vi "Set Inertia Matrix as 1D Array.vi"(8 "error in (no error)":errorcluster, 10 "Inertia":dbl[](array[numeric]), 11 "Link in":refnum<class "Link.lvclass">) -> (0 "error out":errorcluster, 3 "Link out":refnum<class "Link.lvclass">)   [LabVIEW 2013, in "Link.lvclass"]
uses:
  Link.lvclass
  Link.lvclass/Link.ctl
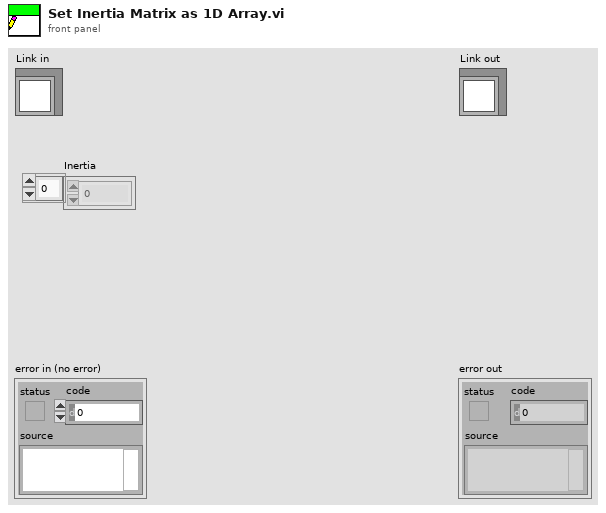
[diagram p1: front panel]
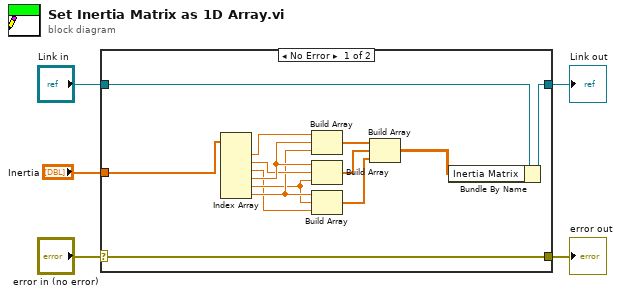
[diagram p0: block diagram]
diagram:
  n1 = case shown="No Error" "error in (no error)" {
    selector: "error in (no error)" -> [w19 w20]
    tunnel: [w19 w20] -> w4
    tunnel: [w17 w21] -> w2
    tunnel: "Link in" -> [w18 w21]
    tunnel: "Inertia" -> [w7 _]
    frame No Error {
      n2 = Index Array(array=w7) -> (element #1=w16:dbl, element #2=w14:dbl, element #3=w11:dbl, element #4=w15:dbl, element #5=w12:dbl, element #6=w13:dbl)  [unwired: 6 in]
      n3 = Build Array(w16, w15, w13) -> (w10:dbl[])
      n4 = Build Array(w15, w14, w12) -> (w9:dbl[])
      n5 = Build Array(w13, w12, w11) -> (w8:dbl[])
      n6 = Build Array(w10, w9, w8) -> (w6:dbl[][])
      n7 = Bundle By Name(cluster=w18, "Inertia Matrix"=w6) -> (w17:refnum<class "Link.lvclass">)
    }
    frame Error {
    }
  }
  "error out" <- w4
  "Link out" <- w2
